vi "PS35_Stop.vi"(2 "error in (no error)":errorcluster, 3 "Axis number":i32=1 min=1 max=3, 4 "Control unit ID":i32=1 min=1 max=10) -> (0 "error out":errorcluster)   [LabVIEW 2020]
doc: "PS35_Stop.vi, created: 04.03.2009 alex; last change: 22.10.2019 alex;\n\n<B>FUNCTION:</B> \n\nStop movement of an axis.\nAny active movement of an axis is terminated. The axis is stopped\nwith the programmed brake ramp and stands still.\n----------------------------------------------------------------------------------------\n<B>INPUT:</B>\n[I32] <B>Control unit ID:</B> control unit index. (Default=1, Range=1...10) \n[I32] <B>Axis number:</B> axis number. (Default=1, Range=1...3) \n[CLU] <B>error in</B>\n----------------------------------------------------------------------------------------\n<B>OUTPUT:</B>\n[CLU] <B>error out</B>\n----------------------------------------------------------------------------------------\n<B>SUB-VIs:</B>\n----------------------------------------------------------------------------------------\n<B>EXT-Calls:</B>\nps35.dll (V2.01)\n----------------------------------------------------------------------------------------"
uses:
  <vilib>/Utility/error.llb/DialogType.ctl
  ps35.dll
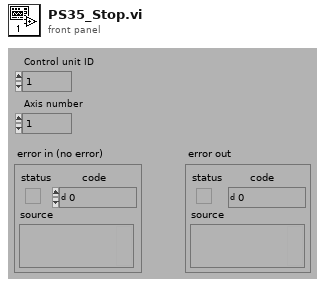
[diagram p1: front panel]
types:
  T1 = typedef "DialogType.ctl" = u16
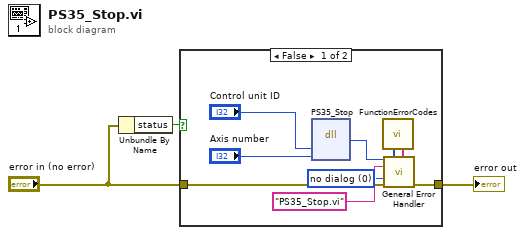
[diagram p0: block diagram]
diagram:
  n1 = Unbundle By Name("error in (no error)") -> ("status"=w1:bool)
  n2 = case shown="False" w1 {
    tunnel: "error in (no error)" -> [w11 w13]
    tunnel: [w10 w13] -> w3
    frame False {
      w4 = T1 0 items=["no dialog", "OK message", "continue or stop message", "OK message + warnings", "continue/stop + warnings"] ("type of dialog (OK msg:1)")
      n3 = dll-call lib="C:/GEECS/Developers Version/source/Device Drivers/OwiSoft_PS35/OWISoftOEM/ps35/labview/lv82/ps35.dll" fn="PS35_Stop"("Index"="Control unit ID", "AxisNr"="Axis number") -> ("Rückgabetyp"=w9:i32)  [unwired: 5 in, 2 out]
      n4 = call "FunctionErrorCodes.vi"() -> ("[user-defined codes]"=w5:i32[], "[user-defined descriptions]"=w6:string[])  [unwired: 8 in]
      n5 = call <vilib>:"General Error Handler.vi"("[error code] (0)"=w9, "[user-defined codes]"=w5, "[user-defined descriptions]"=w6, "[error source] (\" \")"="PS35_Stop.vi" ("[error source] (\" \")"), "type of dialog (OK msg:1)"=w4, "error in (no error)"=w11) -> ("error out"=w10:errorcluster)  [unwired: 5 in, 4 out]
    }
    frame True {
    }
  }
  "error out" <- w3
